vi "3.vi"(8 "Error In":errorcluster) -> (0 "Error Out":errorcluster)   [LabVIEW 2017, in "ErrorStructureDrawer-Tests.lvlib"]
uses:
  ErrorStructureDrawer-Tests.lvlib
panel:
  in  "asfasdfasdf":dbl
  in  "x 2":dbl
  out "x*y":dbl
  in  "x":dbl
  in  "y":dbl
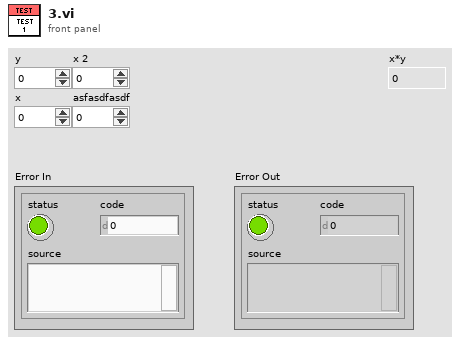
[diagram p1: front panel]
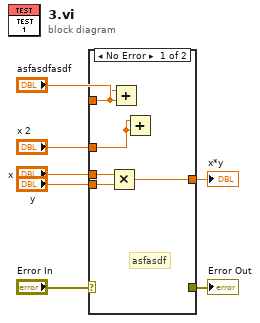
[diagram p0: block diagram]
diagram:
  n1 = case shown="No Error" "Error In" {
    selector: "Error In" -> [_ w13]
    tunnel: "y" -> [w12 _]
    tunnel: "x" -> [w11 _]
    tunnel: [w10 _] -> w5
    tunnel: "x 2" -> [w9 _]
    tunnel: "asfasdfasdf" -> [w8 _]
    tunnel: [_ w13] -> w1
    frame No Error {
      # "asfasdf"
      n2 = Multiply(x=w11, y=w12) -> (x*y=w10:dbl)
      n3 = Add(x=w8, y=w8) -> ()  [unwired: 1 out]
      n4 = Add(x=w9, y=w9) -> ()  [unwired: 1 out]
    }
    frame Error {
    }
  }
  "x*y" <- w5
  "Error Out" <- w1
